vi "matlabAOwffromparam.vi"(0 "Cluster":T1) -> (1 "Waveform":waveform(dbl), 2 "wfsize":i32)   [LabVIEW 2015]
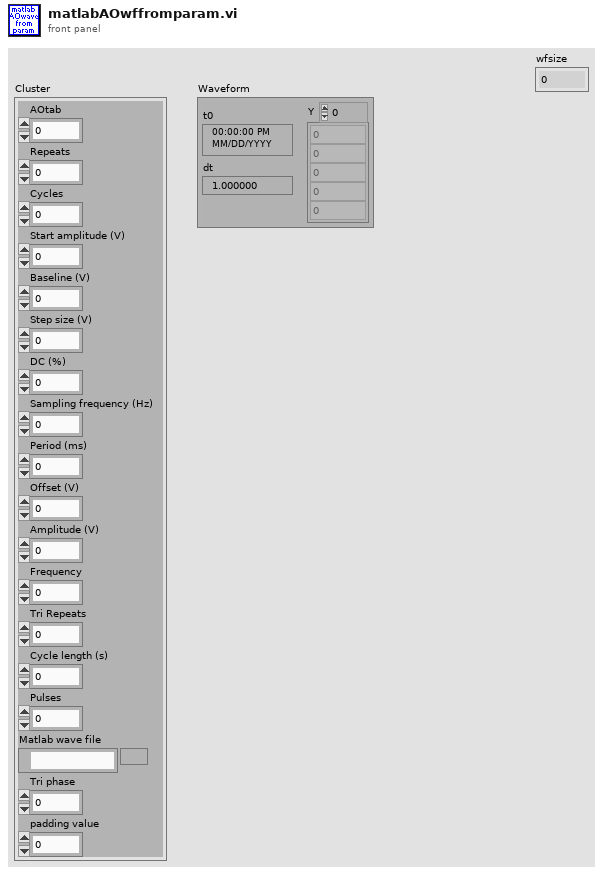
[diagram p1: front panel]
types:
  T1 = cluster{"AOtab":dbl, "Repeats":dbl, "Cycles":dbl, "Start amplitude (V)":dbl, "Baseline (V)":dbl, "Step size (V)":dbl, "DC (%)":dbl, "Sampling frequency (Hz)":dbl, "Period (ms)":dbl, "Offset (V)":dbl, "Amplitude (V)":dbl, "Frequency":dbl, "Tri Repeats":dbl, "Cycle length (s)":dbl, "Pulses":dbl, "Matlab wave file":path, "Tri phase":dbl, "padding value":dbl}
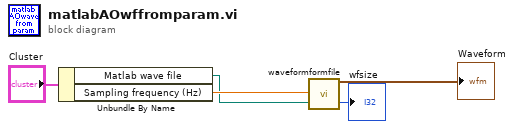
[diagram p0: block diagram]
diagram:
  n1 = Unbundle By Name("Cluster") -> ("Matlab wave file"=w4:path, "Sampling frequency (Hz)"=w5:dbl)
  n2 = call "waveformformfile.vi"("Matlab wave file"=w4, "Sampling frequency (Hz)"=w5) -> ("wfsize"=→"wfsize":i32, "Waveform"=→"Waveform":waveform(dbl))
